vi "globalVariable.vi"() -> ()   [LabVIEW 2020]
panel:
  in  "newTheta3CP":dbl=-78.5639
  in  "newtheta2CP":dbl=-78.5639
  in  "newTheta1CP":dbl=-78.5639
  in  "theta3CP":dbl=-78.5639
  in  "theta2CP":dbl=-78.5639
  in  "theta1CP":dbl=-78.5639
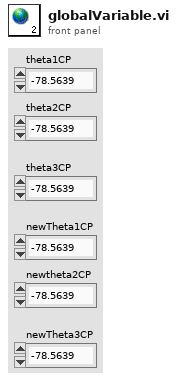
[diagram p1: front panel]
diagram:
